vi "_Open.vi"(8 "error in":errorcluster, 10 "Timeout (mSec)":i32=5000, 11 "Device In":u64) -> (0 "error out":errorcluster, 3 "Device Out":u64)   [LabVIEW 2012, in "Phidget Common.lvlib"]
doc: "Opens a Public"
uses:
  <instrlib>/Phidgets/Phidget Common/Phidget Common.lvlib
  phidget22.dll
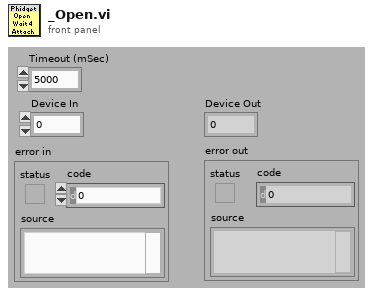
[diagram p1: front panel]
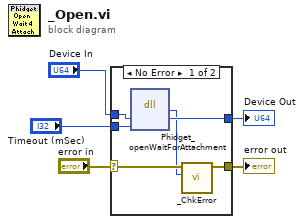
[diagram p0: block diagram]
diagram:
  n1 = case shown="No Error" "error in" {
    selector: "error in" -> [w9 w13]
    tunnel: [w7 w13] -> w4
    tunnel: [w11 w12] -> w3
    tunnel: "Device In" -> [w10 w12]
    tunnel: "Timeout (mSec)" -> [w6 _]
    frame No Error {
      n2 = dll-call lib="phidget22.dll" fn="Phidget_openWaitForAttachment"("phid"=w10, "millis"=w6) -> ("return type"=w8:i32, "phid"=w11:u64)  [unwired: 4 in, 2 out]
      n3 = call <instrlib>:"_ChkError.vi"("Return Code"=w8, "error in (no error)"=w9) -> ("error out"=w7:errorcluster)  [unwired: 9 in]
    }
    frame Error {
    }
  }
  "error out" <- w4
  "Device Out" <- w3
